vi "Read Analogue.vi"(8 "error in (no error)":errorcluster, 11 "Keysight 5700C in":refnum<class "Keysight 5700C.lvclass">) -> (0 "error out":errorcluster, 2 "Measurements":dbl, 3 "Keysight 5700C out":refnum<class "Keysight 5700C.lvclass">)   [LabVIEW 2019, in "Concrete.lvlib" / "Keysight 5700C.lvclass"]
uses:
  Keysight 5700C.lvclass
  Keysight 5700C.lvclass/Keysight 5700C.ctl
  Harware Abstraction/Analog out/Analog out.lvclass
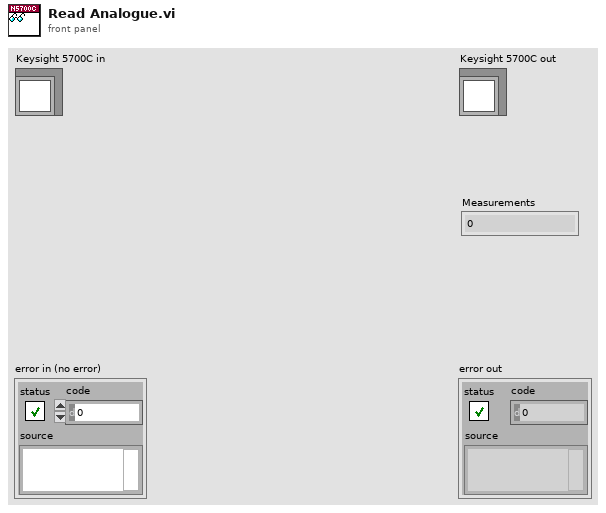
[diagram p1: front panel]
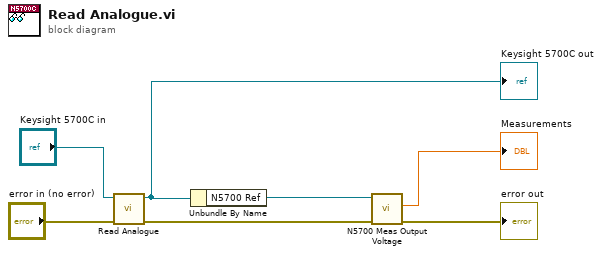
[diagram p0: block diagram]
diagram:
  n1 = call-parent "Read Analogue.vi"("error in (no error)"="error in (no error)", "Analog out in"="Keysight 5700C in") -> ("error out"=w3:errorcluster, "Analog out out"=w5:refnum<class "Keysight 5700C.lvclass">)  [unwired: 7 in, 1 out]
  "Keysight 5700C out" <- w5
  n2 = Unbundle By Name(w5) -> ("N5700 Ref"=w4:refnum<visa-resource-name>)
  n3 = call <instrlib>:"N5700 Meas Output Voltage.vi"("error"=w3, "VISA"=w4) -> ("error out"=→"error out":errorcluster, "Output Voltage"=→"Measurements":dbl)  [unwired: 4 in, 1 out]
